vi "FPGA DDS SineGen IP.vi"(7 "Reset Accumulator":bool, 9 "Signal Amplitude (x 2^15)":u16=32768, 10 "Phase Shift":u32, 11 "Accumulator Increment":u32=100000) -> (2 "Accumulator Value":u32 format="%.3e", 3 "Signal Value":i16)   [LabVIEW 2013]
doc: "This VI generates the next point on a DDS generated sine wave.\n\nThe accumulator increments to calculate the next phase value in the waveform. By varying the accumulator increment you control the frequency of the sine wave.\n\nThe accumulator phase value is used to select a value from the sine wave reference waveform stored in the Lookup Table VI. The waveformcan be p[hase shifted by specifying a non-zero phase shift value which is added to the accumulator phase. The output from the LUT is scaled using the AO Amplitude value."
uses:
  <vilib>/rvi/Arithmetic/AddSubMult/XNode/nirviSatArithmetic.xnode
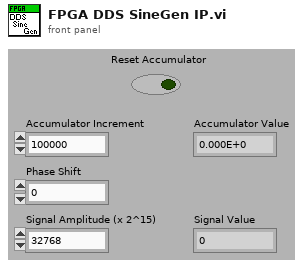
[diagram p1: front panel]
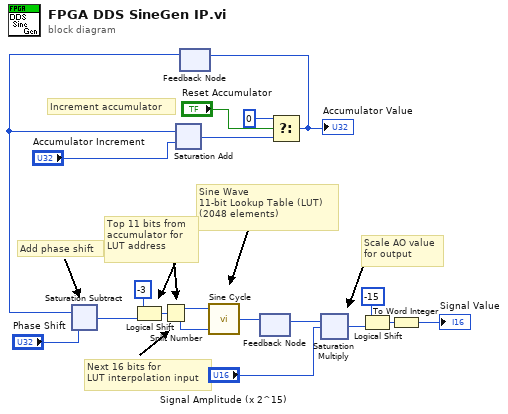
[diagram p0: block diagram]
diagram:
  # "Add phase shift"
  # "Increment accumulator"
  # "Scale AO value\nfor output"
  # "Next 16 bits for\nLUT interpolation input"
  # "Top 11 bits from \naccumulator for\nLUT address"
  # "Sine Wave \n11-bit Lookup Table (LUT)\n(2048 elements)"
  n1 = feedback #1() -> (w3:u32)  [unwired: 1 in]
  n2 = xnode "Saturation Subtract"("x"=w3, "y"="Phase Shift") -> ("x-y"=w2:u32)
  n3 = Logical Shift(y=-3, x=w2) -> (x << y=w12:u32)
  n4 = Split Number(x=w12) -> (hi(x)=w13:u16, lo(x)=w14:u16)
  n5 = xnode ("Saturation Add")("x"=w3, "y"="Accumulator Increment") -> ("x+y"=w9:u32)
  n6 = call "Sine Cycle"("address"=w13, "fractional index (x 2^16)"=w14) -> ("data out"=w15:i16)  [unwired: 7 in]
  n7 = feedback-in #2(w15) -> ()
  n8 = feedback #2() -> (w1:i16)  [unwired: 1 in]
  n9 = Select(t=u32 0, s="Reset Accumulator", f=w9) -> (s? t:f=w11:u32)
  "Accumulator Value" <- w11
  n10 = feedback-in #1(w11) -> ()
  n11 = xnode ("Saturation Multiply")("x"=w1, "y"="Signal Amplitude (x 2^15)") -> ("x*y"=w17:i32)
  n12 = Logical Shift(y=-15, x=w17) -> (x << y=w19:i32)
  n13 = To Word Integer(number=w19) -> (16bit integer=→"Signal Value":i16)
